vi "Read 3D Surface Proprty Array.vi"(8 "error in (no error)":errorcluster, 11 "3D Surface.lvclass in":refnum<class "3D Surface.lvclass">) -> (0 "error out":errorcluster, 2 "3D Surface Proprty Array":T1, 3 "3D Surface.lvclass out":refnum<class "3D Surface.lvclass">)   [LabVIEW 2020, in "3D Surface.lvclass"]
uses:
  3D Surface.lvclass
  3D Surface Property Array.ctl
  3D Surface Property.ctl
  Color Ramp Cluster.ctl
  Line Type.ctl
  3D Surface.lvclass/3D Surface.ctl
  3D Plot.lvclass
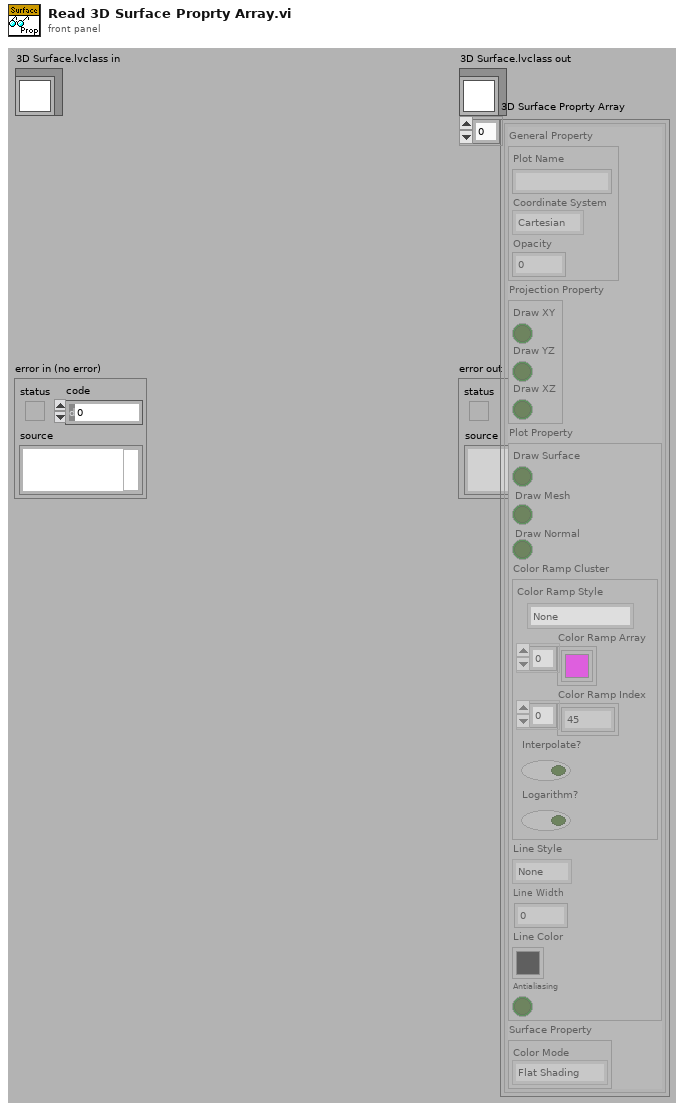
[diagram p1: front panel]
types:
  T1 = typedef "3D Surface.lvclass/3D Surface Property Array.ctl" = T2[]
  T2 = typedef "3D Surface.lvclass/3D Surface Property.ctl" = cluster{"General Property":cluster{"Plot Name":string, "Coordinate System":enum16{"Cartesian", "Cylindrical", "Spherical"}, "Opacity":sgl}, "Projection Property":cluster{"Draw XY":bool, "Draw YZ":bool, "Draw XZ":bool}, "Plot Property":cluster{"Draw Surface":bool, "Draw Mesh":bool, "Draw Normal":bool, "Color Ramp Cluster":T3, "Line Style":T4, "Line Width":sgl, "Line Color":u32, "Antialiasing":bool}, "Surface Property":cluster{"Color Mode":enum16{"Flat Shading", "Interpolated Shading"}}}
  T3 = typedef "3D Plot.lvclass/Color Ramp Cluster.ctl" = cluster{"Color Ramp Style":enum16{"None", "Shaded", "Color spectrum", "Grey scale", "Custom"}, "Color Ramp Array":u32[], "Color Ramp Index":i32[], "Interpolate?":bool, "Logarithm?":bool}
  T4 = typedef "3D Plot.lvclass/Line Type.ctl" = enum16{"None", "Solid", "Dash", "Dot", "Dash Dot"}
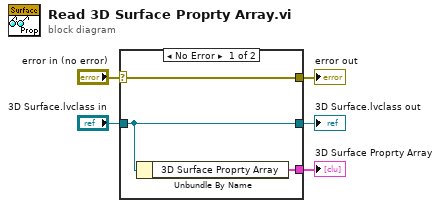
[diagram p0: block diagram]
diagram:
  n1 = case shown="No Error" "error in (no error)" {
    selector: "error in (no error)" -> [w8 w9]
    tunnel: [w8 w9] -> w4
    tunnel: [w7 w10] -> w2
    tunnel: "3D Surface.lvclass in" -> [w7 w10]
    tunnel: [w6 _] -> w1
    frame No Error {
      n2 = Unbundle By Name(w7) -> ("3D Surface Proprty Array"=w6:T1)
    }
    frame Error {
    }
  }
  "error out" <- w4
  "3D Surface.lvclass out" <- w2
  "3D Surface Proprty Array" <- w1
